vi "DCPowerInstrument_CallCreateSessionWithUnregisteredSessionReserved_RemoteSessionCreated.vi"(8 "error in":errorcluster) -> (0 "error out":errorcluster, 2 "result":string, 3 "pass":bool)   [LabVIEW 2020, in "MeasurementServerTests.lvlib"]
uses:
  MeasurementServerTests.lvlib
  Runtime/MeasurementLink niDCPower/Create Sessions - 1Sess.vi
  Runtime/MeasurementLink Session Management/Session Reservation/Session Reservation.lvclass
  Runtime/MeasurementLink niDCPower/MeasurementLink niDCPower.lvlib
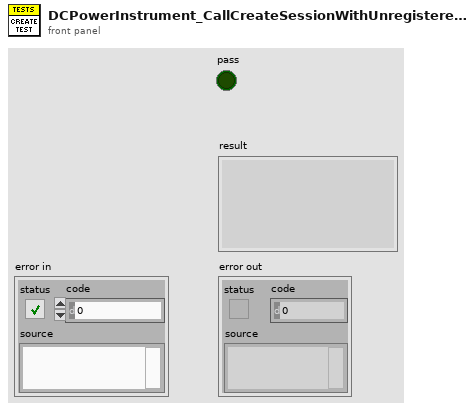
[diagram p1: front panel]
types:
  T1 = typedef "MeasurementLink Session Management.lvlib/Session Reservation.lvclass/Data.ctl" = cluster{"session and driver infos":T2[], "pin or relay names":string[]}
  T2 = typedef "MeasurementLink Session Management.lvlib/Session Reservation.lvclass/Session and Driver Info.ctl" = cluster{"session info":T3, "session":variant}
  T3 = typedef "MeasurementLink Session Management Client.lvlib/ni_measurementlink_sessionmanagement_v1_SessionInformation.ctl" = cluster{"session":T4, "resource_name":string, "channel_list":string, "instrument_type_id":string, "session_exists":bool, "channel_mappings":T5[]}
  T4 = typedef "MeasurementLink Session Management Client.lvlib/nidevice_grpc_Session.ctl" = cluster{"name":string}
  T5 = typedef "MeasurementLink Session Management Client.lvlib/ni_measurementlink_sessionmanagement_v1_ChannelMapping.ctl" = cluster{"pin_or_relay_name":string, "site":i32, "channel":string}
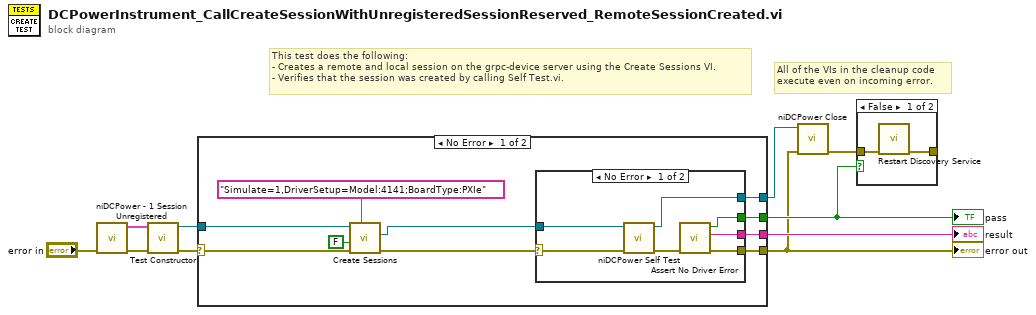
[diagram p0: block diagram]
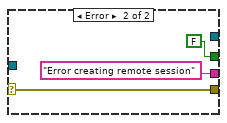
[diagram p2: hidden frame]
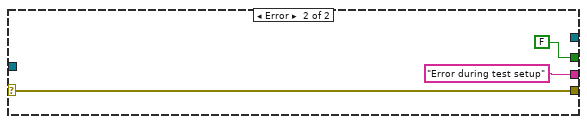
[diagram p3: hidden frame]
diagram:
  # "All of the VIs in the cleanup code\nexecute even on incoming error."
  # "This test does the following:\n- Creates a remote and local session on the grpc-device server using the Create Sessions VI.\n- Verifies that the session was created by calling Self Test.vi."
  n1 = call "niDCPower - 1 Session Unregistered.vi"("error in"="error in") -> ("error out"=w4:errorcluster, "data out"=w5:T1)  [unwired: 9 in]
  n2 = call "Test Constructor.vi"("error in"=w4, "data"=w5) -> ("error out"=w2:errorcluster, "Session Reservation out"=w1:refnum<class "Session Reservation.lvclass">)  [unwired: 8 in]
  n3 = case shown="No Error" w2 {
    selector: w2 -> [w15 w31]
    tunnel: [w19 w31] -> w6
    tunnel: [w20 FALSE] -> w7
    tunnel: [w18 "Error during test setup" ("f")] -> w10
    tunnel: [w17 _] -> w9
    tunnel: w1 -> [w16 _]
    frame No Error {
      n4 = call-poly "Create Sessions.vi"("option string"="Simulate=1,DriverSetup=Model:4141;BoardType:PXIe", "error in"=w15, "reset"=FALSE, "session reservation in"=w16) -> ("error out"=w12:errorcluster, "session"=w11:refnum<k15>)  [unwired: 4 in, 2 out]
      n5 = case shown="No Error" w12 {
        selector: w12 -> [w21 w29]
        tunnel: [w27 FALSE] -> w20
        tunnel: [w25 w29] -> w19
        tunnel: [w26 "Error creating remote session"] -> w18
        tunnel: [w24 _] -> w17
        tunnel: w11 -> [w22 _]
        frame No Error {
          n6 = call <instrlib>:"niDCPower Self Test.vi"("error in (no error)"=w21, "instrument handle"=w22) -> ("error out"=w23:errorcluster, "instrument handle out"=w24:refnum<k15>)  [unwired: 6 in, 2 out]
          n7 = call "Assert No Driver Error.vi"("error in"=w23) -> ("error out"=w25:errorcluster, "result"=w26:string, "pass?"=w27:bool)  [unwired: 8 in]
        }
        frame Error {
        }
      }
    }
    frame Error {
    }
  }
  "error out" <- w6
  "pass" <- w7
  "result" <- w10
  n8 = call <instrlib>:"niDCPower Close.vi"("error in (no error)"=w6, "instrument handle"=w9) -> ("error out"=w8:errorcluster)  [unwired: 9 in]
  n9 = case shown="False" w7 {
    tunnel: w8 -> [w35 _]
    tunnel: [w34 _] -> _
    frame False {
      n10 = call "Restart Discovery Service.vi"("error in"=w35) -> ("error out"=w34:errorcluster)  [unwired: 10 in]
    }
    frame True {
    }
  }
